vi "HR Humidity Ration of Humid Air(Kg to Kg).vi"(1 "Gas Presure":dbl[unit]=80000.0 min=80000.0 max=120000.0, 2 "Tceg":dbl[unit], 3 "RH":dbl) -> (0 "HR":dbl)   [LabVIEW 2018]
panel:
  out "HR\nPressure of Humid Air Humidity Ratio(Kg/Kg)\nHR=PDWV/PDDA":dbl(knob) scale=0.0..5.0
  out "Temprature Of Input Air\nKelvin Degree":dbl[unit](slide) scale=273.0..373.0
  out "Tk":dbl[unit]
  out "Temprature Of Input Air\nCentigrade Degree":dbl[unit](slide) scale=0.0..100.0
  out "Humidity of Input Air":dbl(knob) scale=0.0..100.0
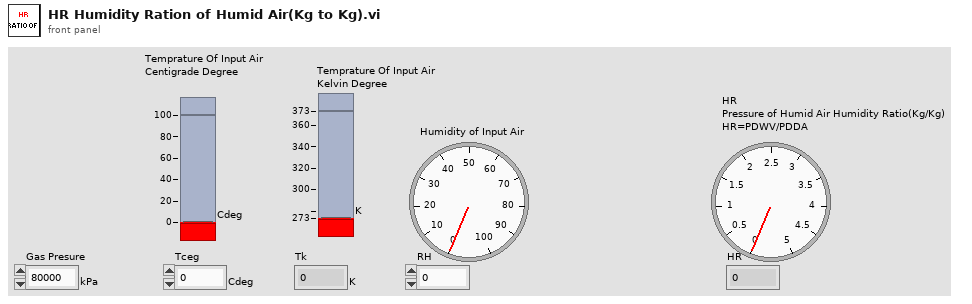
[diagram p1: front panel]
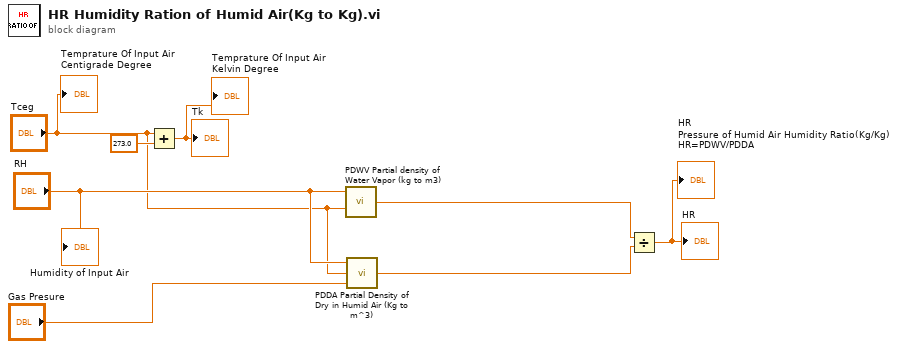
[diagram p0: block diagram]
diagram:
  n1 = Add(x="Tceg", y=dbl[unit] 273.0) -> (x+y=→"Tk" →"Temprature Of Input Air\nKelvin Degree":dbl[unit])
  n2 = call "PDWV Partial density of Water Vapor (kg to m3).vi"("Tceg"="Tceg", "RH"="RH") -> ("PDWV"=w5:dbl[unit])
  n3 = call "PDDA Partial Density of Dry in Humid Air (Kg to m^3).vi"("Total Pressure of Humid Air"="Gas Presure", "Tceg"="Tceg", "RH"="RH") -> ("PDDA"=w4:dbl[unit])
  n4 = Divide(x=w5, y=w4) -> (x/y=→"HR\nPressure of Humid Air Humidity Ratio(Kg/Kg)\nHR=PDWV/PDDA" →"HR":dbl)
  "Humidity of Input Air" <- "RH"
  "Temprature Of Input Air\nCentigrade Degree" <- "Tceg"
